vi "icon_from_tag.vi"(8 "error in (no error)":errorcluster, 11 "Tag in":variant) -> (0 "error out":errorcluster, 3 "Icon":picture)   [LabVIEW 2020]
uses:
  <vilib>/LabVIEW Icon API/lv_icon/Classes/Load_Unload/Load & Unload.lvclass
  <vilib>/LabVIEW Icon API/lv_icon/Classes/Icon Framework/Icon Framework.lvclass
  C:/Program Files/National Instruments/LabVIEW 2025/vi.lib/LabVIEW Icon API/lv_icon/Classes/Layer/Layer.lvclass
  <vilib>/LabVIEW Icon API/lv_icon/Classes/Icon/Icon.lvclass
  <vilib>/LabVIEW Icon API/LabVIEW Icon API.lvlib
  <vilib>/LabVIEW Icon API/lv_icon/lv_icon.lvlib
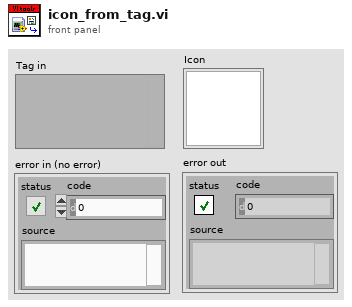
[diagram p1: front panel]
types:
  T1 = cluster{"Layer Name":string, "Color":cluster{"image type":i32, "image depth":i32, "image":u8[], "mask":u8[], "colors":u32[], "Rectangle":cluster{"left":i16, "top":i16, "right":i16, "bottom":i16}}, "B/W":cluster{"image type":i32, "image depth":i32, "image":u8[], "mask":u8[], "colors":u32[], "Rectangle":cluster{"left":i16, "top":i16, "right":i16, "bottom":i16}}}
  T2 = typedef "LabVIEW Icon Stored Information.ctl" = cluster{"Text Visible?":bool, "Text Opacity":u8, "Templ Visible?":bool, "Templ Opacity":u8, "Relative Path from 1 to 2":path, "Image":picture, "All User Layers":refnum<class "Layer.lvclass">[], "Body Text":T3}
  T3 = typedef "BodyText.ctl" = cluster{"Line 1 text":string, "Line 2 text":string, "Line 3 text":string, "Line 4 text":string, "Line 1 color":u32, "Line 2 color":u32, "Line 3 color":u32, "Line 4 color":u32, "Body Text Spec":cluster{"Font":T4, "Alignment":T5, "Size":u8}, "Center text vertically":bool, "Capitalize Text":bool}
  T4 = typedef "Font.ctl" = string
  T5 = typedef "Alignment.ctl" = u16
  T6 = typedef "Layer.ctl" = cluster{"LayerIcon":picture, "LayerName":string, "Opacity":u8, "Visibility?":bool}
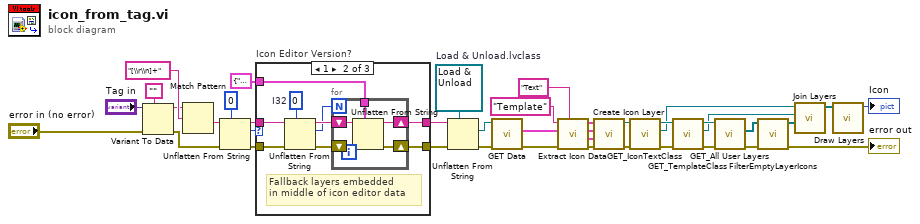
[diagram p0: block diagram]
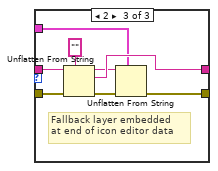
[diagram p3: hidden frame]
diagram:
  w34 = refnum<class "Load & Unload.lvclass"> refnum  # Load & Unload.lvclass
  n1 = Variant To Data(error in="error in (no error)", type="", Variant="Tag in") -> (data=w26:string, error out=w25:errorcluster)
  n2 = Match Pattern(string=w26, regular expression="[\\r\\n]+") -> (after substring=w30:string)  [unwired: 1 in, 3 out]
  n3 = Unflatten From String(type=u8 0 ("U8"), binary string=w30, error in (no error)=w25) -> (rest of the binary string=w29:string, value=w37:u8, error out=w27:errorcluster)  [unwired: 2 in]
  n4 = case "Icon Editor Version?" shown="1" w37 {
    tunnel: w27 -> [w39 w49 w62]
    tunnel: [w39 w45 w57] -> w32
    tunnel: w29 -> [w40 w47 w60]
    tunnel: [w40 w43 w58] -> w33
    tunnel: T1 {"Layer Name"="", "Color"={"image type"=0, "image depth"=0, "image"=[], "mask"=[], "colors"=[], "Rectangle"={"left"=0, "top"=0, "right"=0, "bottom"=0}}, "B/W"={"image type"=0, "image depth"=0, "image"=[], "mask"=[], "colors"=[], "Rectangle"={"left"=0, "top"=0, "right"=0, "bottom"=0}}} ("Fallback Layers") -> [_ w42 w55]
    frame ..0, 3.. {
    }
    frame 1 {
      w46 = 0  # I32
      # "Fallback layers embedded\nin middle of icon editor data"
      n5 = Unflatten From String(type=w46, binary string=w47, error in (no error)=w49) -> (rest of the binary string=w44:string, value=w41:i32, error out=w48:errorcluster)  [unwired: 2 in]
      n6 = for {
        N: w41 -> [_]
        tunnel: w42 -> [w50]
        shift-right: [w53] -> w45
        shift-left: w48 -> [w54]
        shift-right: [w51] -> w43
        shift-left: w44 -> [w52]
        n7 = Unflatten From String(type=w50, binary string=w52, error in (no error)=w54) -> (rest of the binary string=w51:string, error out=w53:errorcluster)  [unwired: 2 in, 1 out]
      }
    }
    frame 2 {
      # "Fallback layer embedded\nat end of icon editor data"
      n8 = Unflatten From String(type="", binary string=w60, error in (no error)=w62) -> (rest of the binary string=w56:string, value=w58:string, error out=w61:errorcluster)  [unwired: 2 in]
      n9 = Unflatten From String(type=w55, binary string=w56, error in (no error)=w61) -> (error out=w57:errorcluster)  [unwired: 2 in, 2 out]
    }
  }
  n10 = Unflatten From String(type=w34, binary string=w33, error in (no error)=w32) -> (value=w36:refnum<class "Load & Unload.lvclass">, error out=w35:errorcluster)  [unwired: 2 in, 1 out]
  n11 = call-dynamic "GET Data.vi"("error in (no error)"=w35, "Load & Unload.lvclass in"=w36) -> ("error out"=w5:errorcluster, "Data"=w16:T2)  [unwired: 7 in, 1 out]
  n12 = call <vilib>:"Extract Icon Data.vi"("Text layer name"="Text", "Icon data in"=w16, "Template layer name"="Template") -> ("Template data"=w19:T6, "Icon data out"=w20:T2, "Text data"=w21:T6)  [unwired: 5 in, 1 out]
  n13 = call <vilib>:"Create Icon Layer.vi"("error in (no error)"=w5, "Template data"=w19, "Icon data"=w20, "Text data"=w21) -> ("error out"=w6:errorcluster, "Icon out"=w7:refnum<class "Icon.lvclass">)  [unwired: 6 in]
  n14 = call-dynamic "GET_IconTextClass.vi"("error in (no error)"=w6, "Icon.lvclass in"=w7) -> ("error out"=w8:errorcluster, "Icon Framework.lvclass"=w11:refnum<class "Icon Framework.lvclass">, "Icon.lvclass out"=w14:refnum<class "Icon.lvclass">)  [unwired: 7 out]
  n15 = call-dynamic "GET_TemplateClass.vi"("error in (no error)"=w8, "Icon.lvclass in"=w14) -> ("error out"=w9:errorcluster, "Icon Framework.lvclass"=w10:refnum<class "Icon Framework.lvclass">, "Icon.lvclass out"=w15:refnum<class "Icon.lvclass">)  [unwired: 7 in]
  n16 = call-dynamic "GET_All User Layers.vi"("error in (no error)"=w9, "Icon.lvclass in"=w15) -> ("error out"=w3:errorcluster, "User Layer"=w4:refnum<class "Layer.lvclass">[])  [unwired: 7 in, 1 out]
  n17 = call <vilib>:"FilterEmptyLayerIcons.vi"("error in (no error)"=w3, "Layers"=w4) -> ("error out"=→"error out":errorcluster, "Layers out"=w12:refnum<class "Layer.lvclass">[])  [unwired: 8 out]
  n18 = call <vilib>:"Join Layers.vi"("User Layers"=w12, "Template"=w10, "Icon Text"=w11) -> ("Layer out"=w13:refnum<class "Layer.lvclass">[])  [unwired: 3 in, 5 out]
  n19 = call <vilib>:"Draw Layers.vi"("Layers"=w13) -> ("Picture"=→"Icon":picture)  [unwired: 4 in, 6 out]
